vi "peakFinding getAnntList.vi"(5 "1stDiffData":dbl[](array[numeric]), 7 "xData":dbl[](array[numeric]), 9 "rightIdx":i32[](array[numeric]), 10 "leftIdx":i32[](array[numeric]), 11 "peakIdx":i32[](array[numeric])) -> (3 "anntList":T1(array[cluster]))   [LabVIEW 2018]
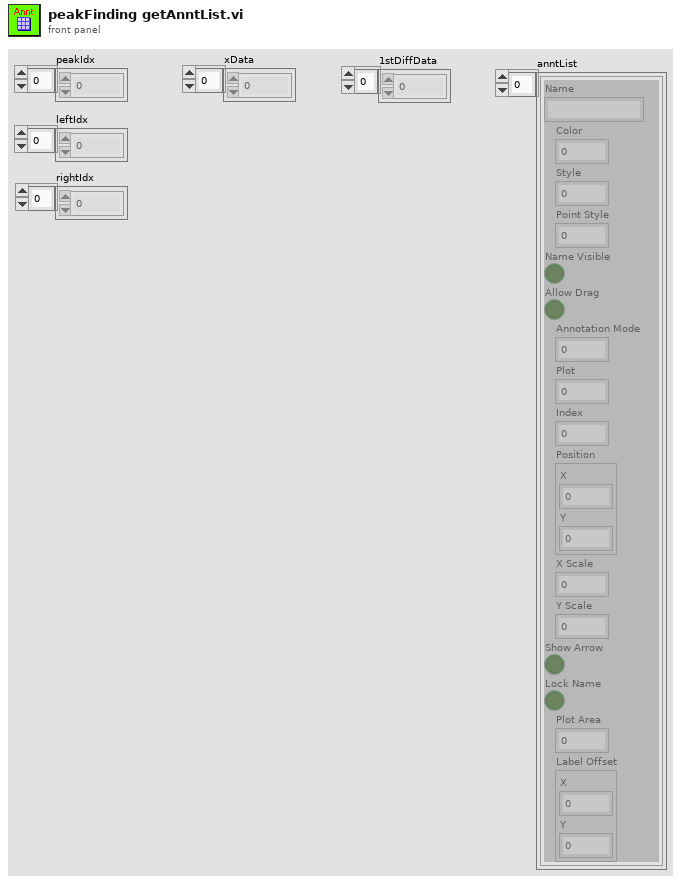
[diagram p1: front panel]
types:
  T1 = cluster{"Name":string, "Color":i32, "Style":u8, "Point Style":i32, "Name Visible":bool, "Allow Drag":bool, "Annotation Mode":u32, "Plot":i32, "Index":i32, "Position":cluster{"X":dbl, "Y":dbl}, "X Scale":u32, "Y Scale":u32, "Show Arrow":bool, "Lock Name":bool, "Plot Area":i32, "Label Offset":cluster{"X":dbl, "Y":dbl}}[]
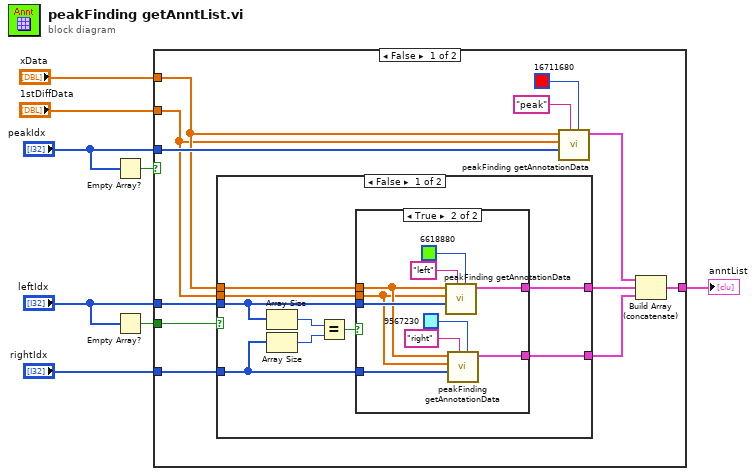
[diagram p0: block diagram]
diagram:
  n1 = Empty Array?(array="peakIdx") -> (empty?=w8:bool)
  n2 = Empty Array?(array="leftIdx") -> (empty?=w6:bool)
  n3 = case shown="False" w8 {
    tunnel: "peakIdx" -> [w17 _]
    tunnel: w6 -> [w20 _]
    tunnel: "leftIdx" -> [w19 _]
    tunnel: "rightIdx" -> [w18 _]
    tunnel: "xData" -> [w14 _]
    tunnel: "1stDiffData" -> [w13 _]
    tunnel: [w9 _] -> w1
    frame False {
      n4 = case shown="False" w20 {
        tunnel: w19 -> [w26 _]
        tunnel: w18 -> [w25 _]
        tunnel: w14 -> [w24 _]
        tunnel: w13 -> [w23 _]
        tunnel: [w22 _] -> w12
        tunnel: [w21 _] -> w10
        frame False {
          n5 = Array Size(array=w26) -> (size(s)=w29:i32)
          n6 = Array Size(array=w25) -> (size(s)=w28:i32)
          n7 = Equal?(x=w29, y=w28) -> (x = y?=w27:bool)
          n8 = case shown="True" w27 {
            tunnel: w26 -> [_ w37]
            tunnel: w25 -> [_ w34]
            tunnel: w24 -> [_ w33]
            tunnel: w23 -> [_ w32]
            tunnel: [_ w31] -> w22
            tunnel: [_ w30] -> w21
            frame False {
            }
            frame True {
              n9 = call "peakFinding getAnnotationData.vi"("Color Box"=u32 6618880, "name"="left", "getIdxArray"=w37, "yData"=w32, "xData"=w33) -> ("AnntData"=w31:T1)  [unwired: 6 in]
              n10 = call "peakFinding getAnnotationData.vi"("Color Box"=u32 9567230, "name"="right", "getIdxArray"=w34, "yData"=w32, "xData"=w33) -> ("AnntData"=w30:T1)  [unwired: 6 in]
            }
          }
        }
        frame True {
        }
      }
      n11 = call "peakFinding getAnnotationData.vi"("Color Box"=u32 16711680, "name"="peak", "getIdxArray"=w17, "yData"=w13, "xData"=w14) -> ("AnntData"=w11:T1)  [unwired: 6 in]
      n12 = Build Array (concatenate)(w11, w12, w10) -> (w9:T1)
    }
    frame True {
    }
  }
  "anntList" <- w1
